vi "Queues.vi"(8 "error in (no error)":errorcluster) -> (0 "error out":errorcluster, 3 "Queues":T1)   [LabVIEW 2021]
uses:
  Typedefs/All_Queues.ctl
  Typedefs/DataToUserInterface.ctl
  Typedefs/PropertyUserChange.ctl
  Typedefs/PropertiesRead_TDM.ctl
  Typedefs/Start_End.ctl
  Typedefs/OrderAnalysis.ctl
  Typedefs/Axis.ctl
  Typedefs/MeassurementMode.ctl
  Typedefs/PropertiesOrderAnalysis.ctl
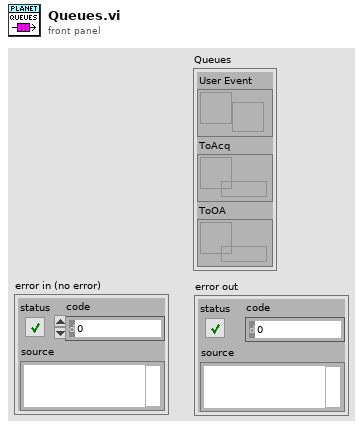
[diagram p1: front panel]
types:
  T1 = typedef "All_Queues.ctl" = cluster{"User Event":refnum<user-event>, "ToAcq":refnum<queue>, "ToOA":refnum<queue>}
  T2 = typedef "PropertiesOrderAnalysis.ctl" = cluster{"Start/End":T3, "data":waveform(dbl)[], "OrderAnalysis":T4, "Tacho":waveform(dbl)[]}
  T3 = typedef "Start_End.ctl" = enum16{"Start", "End"}
  T4 = typedef "OrderAnalysis.ctl" = cluster{"dB on":bool, "window type":u32, "max order to analyze":dbl, "order resolution":dbl, "Axis":T5, "Sample rate":i64, "Save?":bool, "Multiple_Frequency":i32, "averaging mode":enum16{"No averaging", "Vector averaging", "RMS averaging", "Peak hold"}}
  T5 = typedef "Axis.ctl" = u16
  T6 = typedef "PropertiesRead_TDM.ctl" = cluster{"Start/End":T3, "stop":bool, "file path":path, "OrderAnalysis":T4, "Meassurement Mode":T7}
  T7 = typedef "MeassurementMode.ctl" = cluster{"Sample mode":i32, "Terminal conf":i32, "Channels":tag}
  T8 = typedef "DataToUserInterface.ctl" = cluster{"Value":variant, "Property":T9}
  T9 = typedef "PropertyUserChange.ctl" = enum16{"Default", "Results", "Start", "Save", "CanalNames"}
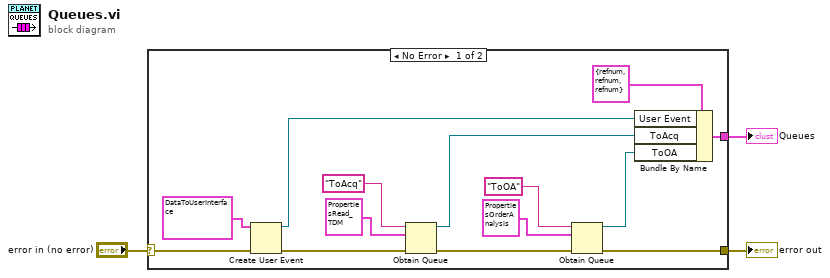
[diagram p0: block diagram]
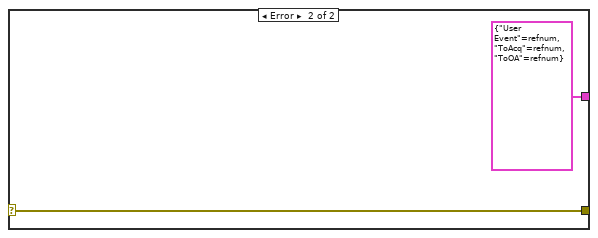
[diagram p2: hidden frame]
diagram:
  n1 = case shown="No Error" "error in (no error)" {
    selector: "error in (no error)" -> [w4 w19]
    tunnel: [w6 w19] -> w3
    tunnel: [w5 T1 {"User Event"=refnum, "ToAcq"=refnum, "ToOA"=refnum} ("Queues")] -> w2
    frame No Error {
      n2 = Create User Event(user event datatype=T8 {"Value"=variant, "Property"=enum."Default"} ("UserData"), error in=w4) -> (user event=w9:refnum<user-event>, error out=w15:errorcluster)
      n3 = Obtain Queue(name (unnamed)="ToAcq", element data type=T6 {"Start/End"=enum."End", "stop"=FALSE, "file path"=path "", "OrderAnalysis"={"dB on"=TRUE, "window type"=1, "max order to analyze"=32.0, "order resolution"=0.1, "Axis"=0, "Sample rate"=5000, "Save?"=FALSE, "Multiple_Frequency"=3, "averaging mode"=enum."No averaging"}, "Meassurement Mode"={"Sample mode"=10123, "Terminal conf"=12529, "Channels"=""}}, error in (no error)=w15) -> (queue out=w8:refnum<queue>, error out=w11:errorcluster)  [unwired: 2 in, 1 out]
      n4 = Obtain Queue(name (unnamed)="ToOA", element data type=T2 {"Start/End"=enum."End", "data"=[], "OrderAnalysis"={"dB on"=TRUE, "window type"=1, "max order to analyze"=32.0, "order resolution"=0.1, "Axis"=0, "Sample rate"=5000, "Save?"=FALSE, "Multiple_Frequency"=3, "averaging mode"=enum."No averaging"}, "Tacho"=[]}, error in (no error)=w11) -> (queue out=w7:refnum<queue>, error out=w6:errorcluster)  [unwired: 2 in, 1 out]
      n5 = Bundle By Name(cluster=T1 {"User Event"=refnum, "ToAcq"=refnum, "ToOA"=refnum} ("Queues"), "User Event"=w9, "ToAcq"=w8, "ToOA"=w7) -> (w5:T1)
    }
    frame Error {
    }
  }
  "error out" <- w3
  "Queues" <- w2
